vi "Init.vi"(6 "Creator Queue":refnum<data-value>, 8 "Creator Queue Alias":string, 9 "Self Queue":refnum<data-value>, 10 "Self Queue Alias":string) -> (3 "Queue Mailbox out":refnum<class "Queue Mailbox.lvclass">)   [LabVIEW 2021, in "jettl.lvlib" / "Queue Mailbox.lvlib" / "Queue Mailbox.lvclass"]
uses:
  Queue Mailbox.lvclass
  Msg Strategy/Msg Strategy.lvclass
  Queue Mailbox.lvclass/Queue Mailbox.ctl
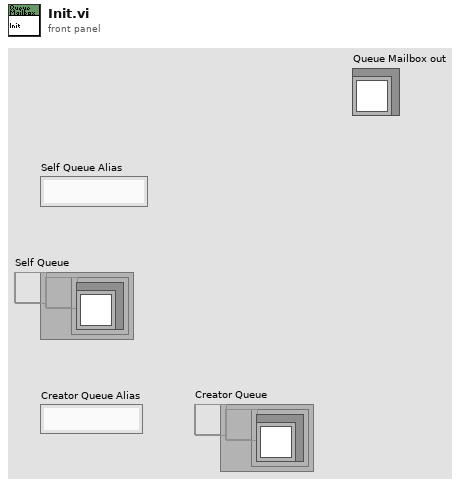
[diagram p1: front panel]
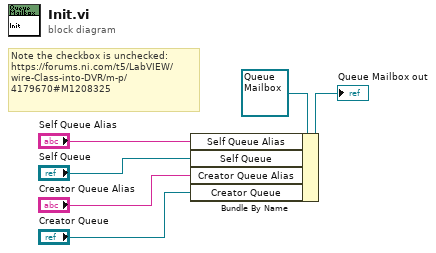
[diagram p0: block diagram]
diagram:
  # "Note the checkbox is unchecked:\nhttps://forums.ni.com/t5/LabVIEW/wire-Class-into-DVR/m-p/4179670#M1208325"
  n1 = Bundle By Name(cluster=refnum<class "Queue Mailbox.lvclass"> refnum ("Queue Mailbox out"), "Self Queue Alias"="Self Queue Alias", "Self Queue"="Self Queue", "Creator Queue Alias"="Creator Queue Alias", "Creator Queue"="Creator Queue") -> (→"Queue Mailbox out":refnum<class "Queue Mailbox.lvclass">)
